vi "DBL to String.vi"(9 "precision (6)":i16, 10 "String":string, 11 "DBL":dbl) -> (2 "number":dbl, 3 "F-format string":string)   [LabVIEW 2021]
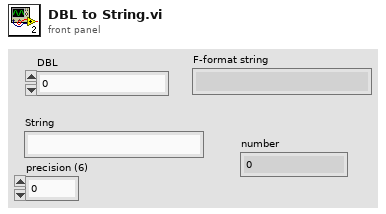
[diagram p1: front panel]
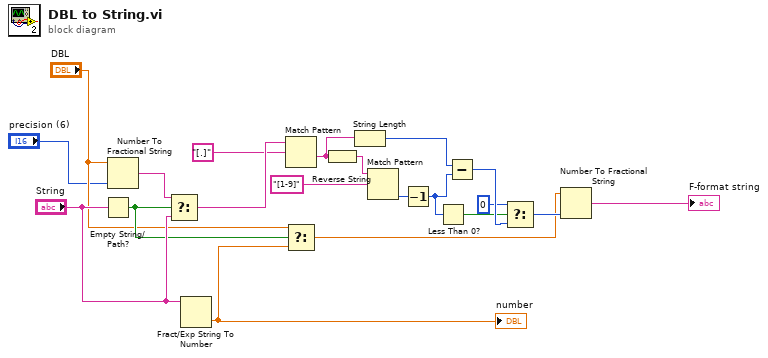
[diagram p0: block diagram]
diagram:
  n1 = Empty String/Path?(string/path="String") -> (empty?=w5:bool)
  n2 = Number To Fractional String(number="DBL", precision (6)="precision (6)") -> (F-format string=w18:string)  [unwired: 2 in]
  n3 = Select(t=w18, s=w5, f="String") -> (s? t:f=w8:string)
  n4 = Fract/Exp String To Number(string="String") -> (number=w4:dbl)  [unwired: 3 in, 1 out]
  "number" <- w4
  n5 = Match Pattern(string=w8, regular expression="[.]") -> (after substring=w11:string)  [unwired: 1 in, 3 out]
  n6 = Select(t="DBL", s=w5, f=w4) -> (s? t:f=w2:dbl)
  n7 = Reverse String(1:w11) -> (0:w10:string)
  n8 = String Length(string=w11) -> (length=w12:i32)
  n9 = Match Pattern(string=w10, regular expression="[1-9]") -> (offset past match=w13:i32)  [unwired: 1 in, 3 out]
  n10 = Decrement(x=w13) -> (x-1=w14:i32)
  n11 = Less Than 0?(x=w14) -> (x < 0?=w16:bool)
  n12 = Subtract(x=w12, y=w14) -> (x-y=w17:i32)
  n13 = Select(t=0, s=w16, f=w17) -> (s? t:f=w6:i32)
  n14 = Number To Fractional String(number=w2, precision (6)=w6) -> (F-format string=→"F-format string":string)  [unwired: 2 in]
